vi "CalcularArea.vi"(8 "error in":errorcluster, 11 "object in":refnum<class "FiguraGeometrica.lvclass">) -> (0 "error out":errorcluster, 2 "Area":dbl, 3 "object out":refnum<class "FiguraGeometrica.lvclass">)   [LabVIEW 2024, in "FiguraGeometrica.lvclass"]
uses:
  FiguraGeometrica.lvclass
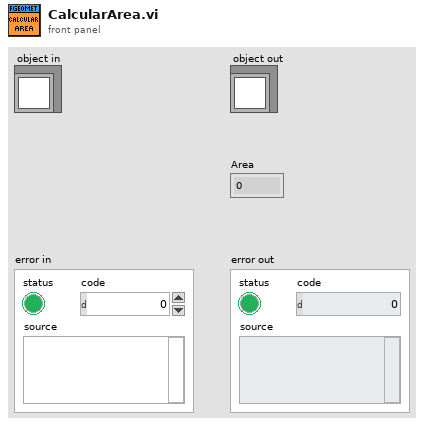
[diagram p1: front panel]
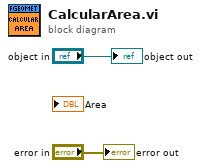
[diagram p0: block diagram]
diagram:
  "error out" <- "error in"
  "object out" <- "object in"
